vi "runTimestampUpdate.vi"(8 "error in (no error)":errorcluster, 11 "Boot in":refnum<class "Boot.lvclass">) -> (0 "error out":errorcluster, 3 "Boot out":refnum<class "Boot.lvclass">)   [LabVIEW 2016, in "Boot.lvclass"]
uses:
  Boot.lvclass
  Boot.lvclass/Boot.ctl
  UserEvents/UserEvents.lvclass/UserEvents.ctl
  Common_RT_Timestamp/Timestamp/Timestamp.lvclass
  UserEvents/UserEvents.lvclass
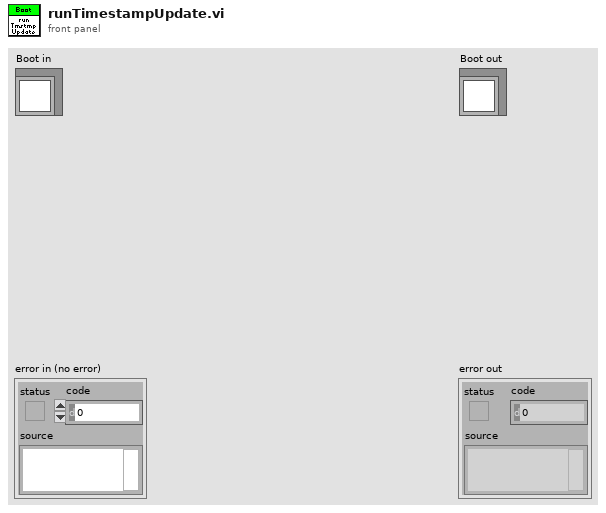
[diagram p1: front panel]
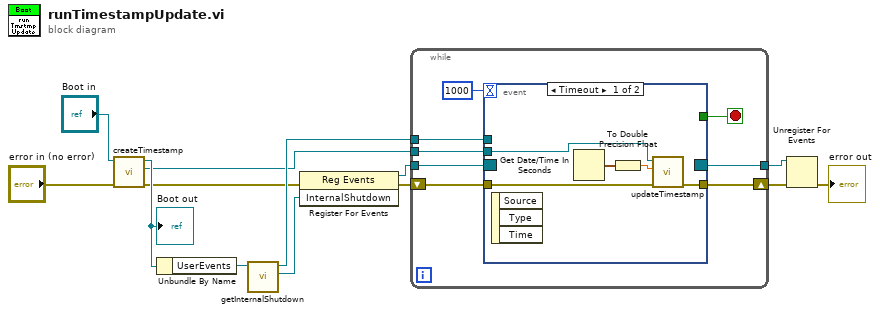
[diagram p0: block diagram]
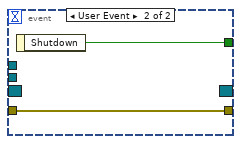
[diagram p2: hidden frame]
diagram:
  n1 = call "createTimestamp.vi"("error in (no error)"="error in (no error)", "Boot in"="Boot in") -> ("error out"=w1:errorcluster, "Timestamp"=w3:refnum<class "Timestamp.lvclass">, "Boot out"=w4:refnum<class "Boot.lvclass">)  [unwired: 7 in]
  "Boot out" <- w4
  n2 = Unbundle By Name(w4) -> ("UserEvents"=w12:refnum<class "UserEvents.lvclass">)
  n3 = call "getInternalShutdown.vi"("UserEvents in"=w12) -> ("InternalShutdown"=w13:refnum<user-event>, "UserEvents out"=w11:refnum<class "UserEvents.lvclass">)  [unwired: 9 in]
  n4 = register-events(error in=w1, w13) -> (reference out=w10:refnum<event-registration>, error out=w9:errorcluster)  [unwired: 1 in]
  n5 = while {
    tunnel: w10 -> [w20]
    tunnel: [w19] -> w7
    tunnel: w11 -> [w17]
    tunnel: w3 -> [w16]
    shift-right: [w14] -> w8
    shift-left: w9 -> [w15]
    stop <- w18 stop-if-true
    n6 = event shown="[0] Timeout" {
      selector: w20 -> [_ _]
      dyn-events: [_ _] -> w19
      timeout: 1000 -> [_ _]
      tunnel: [_ w28] -> w18
      tunnel: w17 -> [_ _]
      tunnel: w16 -> [w26 _]
      tunnel: w15 -> [w23 w27]
      tunnel: [w22 w27] -> w14
      event Timeout {
        n7 = event-data() -> ()  [unwired: 1 in, 3 out]
        n8 = Get Date/Time In Seconds() -> (seconds since 1Jan1904=w25:timestamp)
        n9 = To Double Precision Float(number=w25) -> (double precision float=w24:dbl)
        n10 = call "updateTimestamp.vi"("error in (no error)"=w23, "Timestamp"=w24, "Timestamp in"=w26) -> ("error out"=w22:errorcluster)  [unwired: 7 in, 1 out]
      }
      event User Event {
        n11 = event-data() -> ("Shutdown"=w28:bool)  [unwired: 1 in]
      }
    }
  }
  n12 = Unregister For Events(event registration refnum=w7, error in=w8) -> (error out=→"error out":errorcluster)
